vi "Remove Timer.vi"(8 "error in (no error)":errorcluster, 10 "Timer Config":T1={"Name"="", "Period [s]"=0.0, "Enabled"=TRUE, "Metadata"=""}, 11 "Task Scheduler Actor in":refnum<class "Task Scheduler Actor.lvclass">) -> (0 "error out":errorcluster, 3 "Task Scheduler Actor out":refnum<class "Task Scheduler Actor.lvclass">)   [LabVIEW 2015, in "Task Scheduler Actor.lvclass"]
uses:
  Task Scheduler Actor.lvclass
  Timer Config.ctl
  Task Scheduler Actor.lvclass/Task Scheduler Actor.ctl
  Re-use Libraries/Timer/Timer.lvclass/Timer.ctl
  Re-use Libraries/Timer/Timer.lvclass
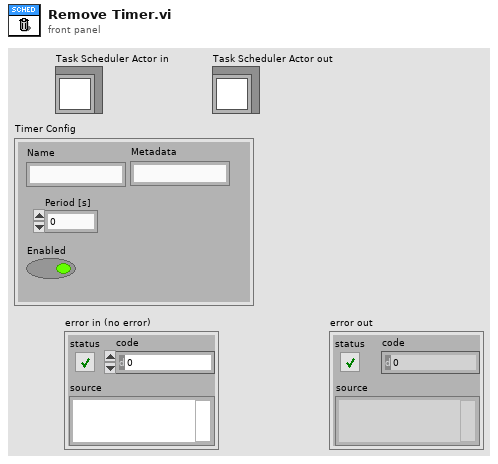
[diagram p1: front panel]
types:
  T1 = typedef "Task Scheduler Actor.lvclass/Timer Config.ctl" = cluster{"Name":string, "Period [s]":dbl, "Enabled":bool, "Metadata":string}
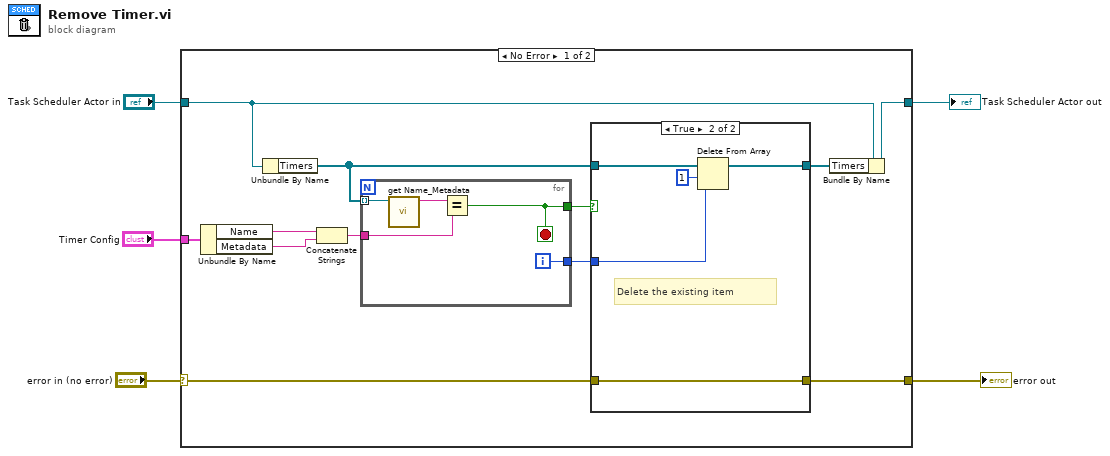
[diagram p0: block diagram]
diagram:
  n1 = case shown="No Error" "error in (no error)" {
    selector: "error in (no error)" -> [w12 w31]
    tunnel: [w17 w30] -> w5
    tunnel: "Task Scheduler Actor in" -> [w16 w30]
    tunnel: "Timer Config" -> [w11 _]
    tunnel: [w13 w31] -> w2
    frame No Error {
      n2 = Unbundle By Name(w11) -> ("Name"=w10:string, "Metadata"=w9:string)
      n3 = Unbundle By Name(w16) -> ("Timers"=w15:refnum<class "Timer.lvclass">[])
      n4 = Concatenate Strings(w10, w9) -> (w8:string)
      n5 = for {
        tunnel: w15 -> [w28] mode=indexing
        tunnel: [w29] -> w14
        tunnel: w8 -> [w26]
        tunnel: [w25] -> w7
        i -> [w25]
        stop <- w29 stop-if-true
        n6 = call "get Name_Metadata .vi"("Timer in"=w28) -> ("Name"=w27:string)  [unwired: 10 in]
        n7 = Equal?(x=w27, y=w26) -> (x = y?=w29:bool)
      }
      n8 = case shown="True" w14 {
        tunnel: w15 -> [w18 w24]
        tunnel: [w18 w23] -> w6
        tunnel: [w19 w22] -> w13
        tunnel: w12 -> [w19 w22]
        tunnel: w7 -> [_ w21]
        frame False {
          # "Not found. Should not really happen but safe just to do nothing"
        }
        frame True {
          # "Delete the existing item"
          n9 = Delete From Array(array=w24, length=1, index=w21) -> (array with subset deleted=w23:refnum<class "Timer.lvclass">[])  [unwired: 1 out]
        }
      }
      n10 = Bundle By Name(cluster=w16, "Timers"=w6) -> (w17:refnum<class "Task Scheduler Actor.lvclass">)
    }
    frame Error {
    }
  }
  "Task Scheduler Actor out" <- w5
  "error out" <- w2
